vi "kostka.vi"() -> ()   [LabVIEW 2022 SP3]
uses:
  <vilib>/numeric/Random Number (Range) U64.vi
  <vilib>/numeric/sub_Random U32.vi
panel:
  in  "stop":bool
  in  "losuj":bool
  out "?":bool
  out "?":bool
  out "?":bool
  out "?":bool
  out "?":bool
  out "?":bool
  out "?":bool
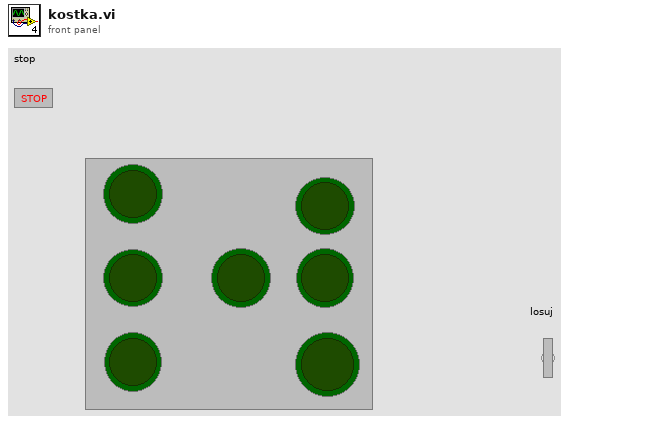
[diagram p1: front panel]
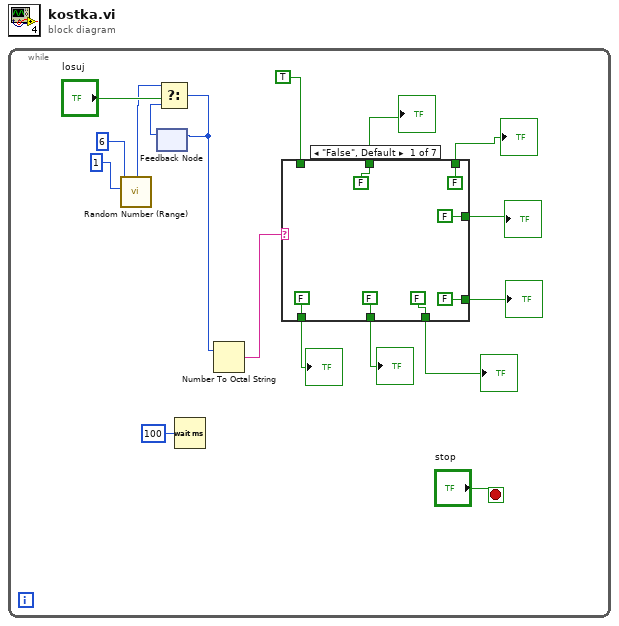
[diagram p0: block diagram]
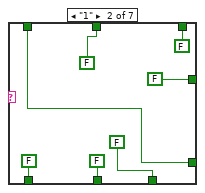
[diagram p2: hidden frame]
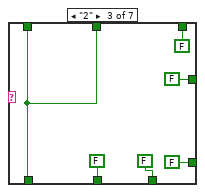
[diagram p3: hidden frame]
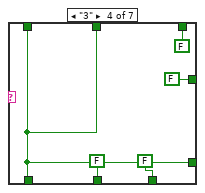
[diagram p4: hidden frame]
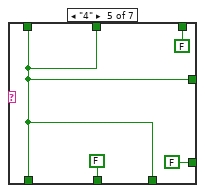
[diagram p5: hidden frame]
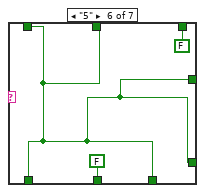
[diagram p6: hidden frame]
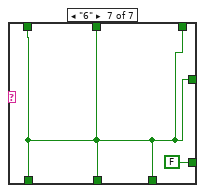
[diagram p7: hidden frame]
diagram:
  n1 = while {
    stop <- "stop" stop-if-true
    n2 = call-poly <vilib>:"Random Number (Range).vi"("lower bound (0)"=u64 1, "upper bound (100)"=u64 6) -> ("number"=w3:u64)  [unwired: 9 in]
    n3 = feedback #1() -> (w1:u64)  [unwired: 1 in]
    n4 = Select(t=w3, s="losuj", f=w1) -> (s? t:f=w2:u64)
    n5 = feedback-in #1(w2) -> ()
    n6 = Wait (ms)(milliseconds to wait=u32 100) -> ()  [unwired: 1 out]
    n7 = Number To Octal String(2:w2) -> (0:w13:string)  [unwired: 1 in]
    n8 = case shown="\"False\", Default" w13 {
      tunnel: [FALSE ("Boolean 8") w31 FALSE ("Boolean 8") w42 FALSE ("Boolean 8") w49 FALSE ("Boolean 8")] -> w12
      tunnel: TRUE ("Boolean 8") -> [_ w31 w36 w42 w46 w49 w51]
      tunnel: [FALSE ("Boolean 8") FALSE ("Boolean 5") FALSE ("Boolean 5") FALSE ("Boolean 8") w46 w49 w51] -> w11
      tunnel: [FALSE ("Boolean 8") FALSE ("Boolean 8") w36 w42 w46 w49 w51] -> w10
      tunnel: [FALSE ("Boolean 8") FALSE ("Boolean 8") FALSE ("Boolean 8") FALSE ("Boolean 8") FALSE ("Boolean 8") FALSE ("Boolean 8") w51] -> w9
      tunnel: [FALSE ("Boolean 8") FALSE ("Boolean 8") FALSE ("Boolean 8") FALSE ("Boolean 8") w46 w49 w51] -> w8
      tunnel: [FALSE ("Boolean 8") FALSE ("Boolean 8") FALSE ("Boolean 8") FALSE ("Boolean 8") FALSE ("Boolean 8") FALSE ("Boolean 8") w51] -> w7
      tunnel: [FALSE ("Boolean 8") FALSE ("Boolean 8") w36 w42 w46 w49 w51] -> w6
      frame "False", Default {
      }
      frame "1" {
      }
      frame "2" {
      }
      frame "3" {
      }
      frame "4" {
      }
      frame "5" {
      }
      frame "6" {
      }
    }
    "?" <- w10
    "?" <- w9
    "?" <- w8
    "?" <- w12
    "?" <- w11
    "?" <- w7
    "?" <- w6
  }
